vi "Adjust To Vision Target.vi"(2 "Y":dbl, 3 "X":dbl) -> (0 "Motor Output":dbl, 1 "Output":bool)   [LabVIEW 2018]
uses:
  <vilib>/addons/control/pid/pid.llb/PID (DBL).vi
  <vilib>/addons/control/pid/NI_PID_pid.lvlib
panel:
  in  "PID Values":cluster{"P":dbl, "I":dbl, "D":dbl}={"P"=0.05, "I"=0.0, "D"=0.0}
  in  "dt":dbl=0.01
  out "Motor Output":dbl
  out "dt output":dbl
  in  "Output Range":cluster{"MAX":dbl, "MIN":dbl}={"MAX"=0.8, "MIN"=-0.8}
  in  "X Image Center":dbl=320.0
  in  "Left Pixel Limit":dbl=300.0
  in  "Right Pixel Limit":dbl=340.0
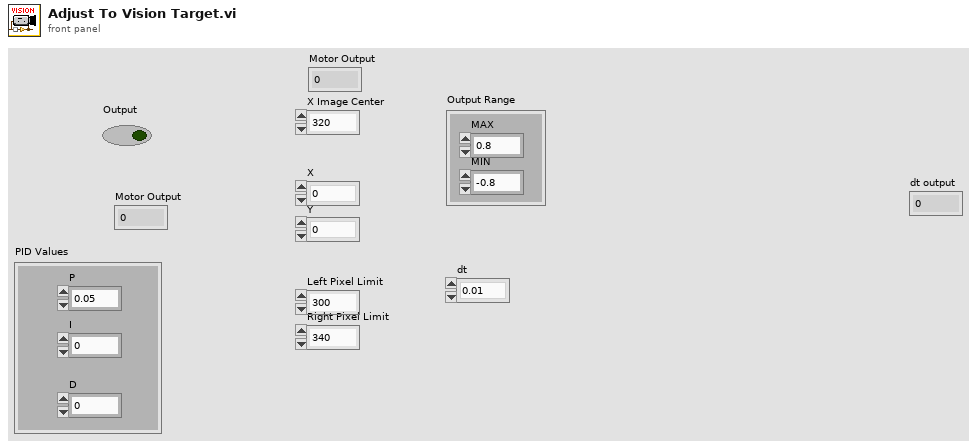
[diagram p1: front panel]
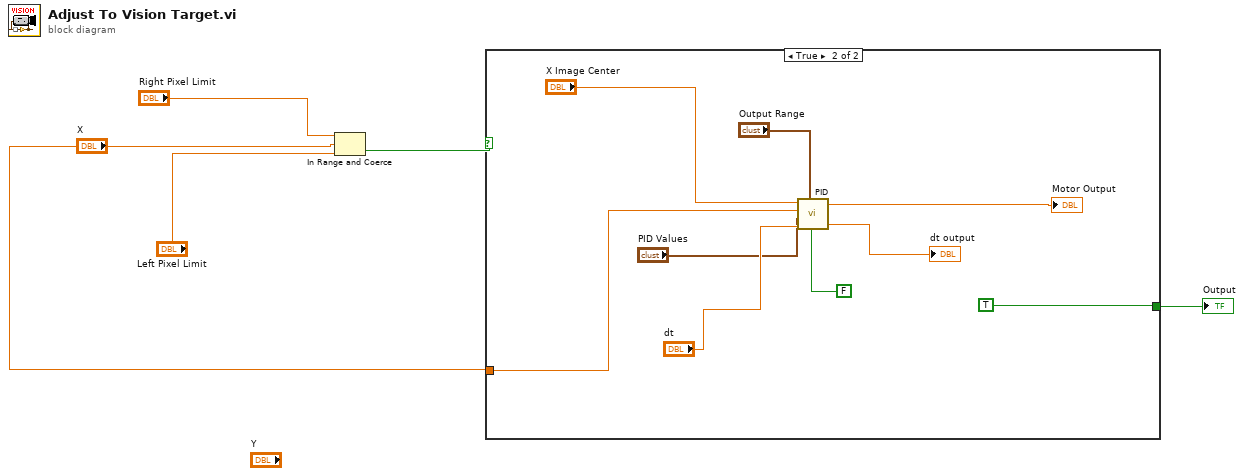
[diagram p0: block diagram]
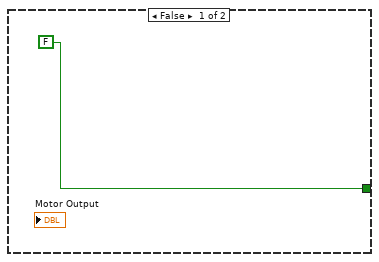
[diagram p2: hidden frame]
diagram:
  n1 = In Range and Coerce(upper limit="Right Pixel Limit", x="X", lower limit="Left Pixel Limit") -> (In Range?=w3:bool)  [unwired: 1 out]
  n2 = case shown="True" w3 {
    tunnel: "X" -> [_ w11]
    tunnel: [FALSE TRUE] -> w1
    frame False {
    }
    frame True {
      n3 = call-poly <vilib>:"PID.vi"("reinitialize? (F)"=FALSE, "output range"="Output Range", "dt (s)"="dt", "PID gains"="PID Values", "process variable"=w11, "setpoint"="X Image Center") -> ("dt out (s)"=→"dt output":dbl, "output"=→"Motor Output":dbl)  [unwired: 4 in]
    }
  }
  "Output" <- w1
